vi "Sample Gun Speed.vi"(10 "Encoder Counts per Rotation":dbl format="%#_13g", 11 "Shooter Rotations":dbl) -> (3 "Shooter RPM":dbl)   [LabVIEW 2015]
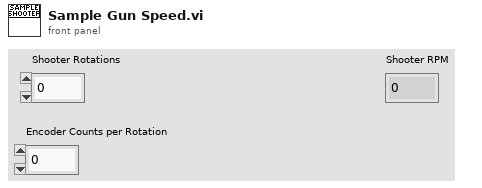
[diagram p1: front panel]
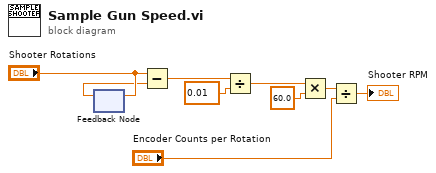
[diagram p0: block diagram]
diagram:
  n1 = feedback-in #1("Shooter Rotations") -> ()
  n2 = feedback #1() -> (w8:dbl)  [unwired: 1 in]
  n3 = Subtract(x="Shooter Rotations", y=w8) -> (x-y=w7:dbl)
  n4 = Divide(x=w7, y=0.01) -> (x/y=w5:dbl)
  n5 = Multiply(x=w5, y=60.0) -> (x*y=w3:dbl)
  n6 = Divide(x=w3, y="Encoder Counts per Rotation") -> (x/y=→"Shooter RPM":dbl)
